vi "beep_pc.vi"(2 "error in":errorcluster, 3 "Duration (seconds)":i32, 4 "Frequency (Hz)":i32) -> (0 "error out":errorcluster)   [LabVIEW 8.6]
doc: "Causes the system to issue an audible tone."
uses:
  kernel32.dll
panel:
  # "See block diagram for instructions."
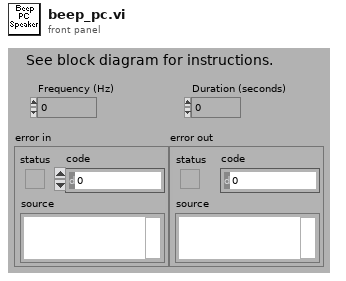
[diagram p1: front panel]
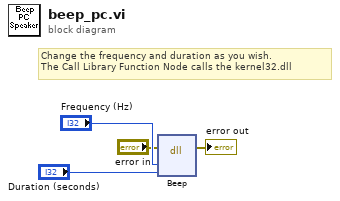
[diagram p0: block diagram]
diagram:
  # "Change the frequency and duration as you wish.\nThe Call Library Function Node calls the kernel32.dll"
  n1 = dll-call lib="KERNEL32.DLL" fn="Beep"(error in="error in", "Frequency (Hz)", "Duration (seconds)") -> (error out=→"error out":errorcluster)  [unwired: 5 in, 1 out]
